vi "Discover Plugins from Loader.vi"(8 "error in (no error)":errorcluster, 10 "Discovery Command":T1, 11 "CIFPluginManager in":refnum<class "CIFPluginManager.lvclass">) -> (0 "error out":errorcluster)   [LabVIEW 2021, in "CIFPluginManager.lvclass"]
uses:
  CIFPluginManager.lvclass
  CIFPluginManager.lvclass/CIFPluginManager.ctl
  CIFCore/Common/Typedef/Version.ctl
  CIFCore/Common/CIFCoreCommon.lvlib
  typedef/Discovered Plugin.ctl
  typedef/Plugin Metadata.ctl
  typedef/Loader Type.ctl
  CIFPluginLoader/gRPC/CIF_Plugin_Loader_Client_Wrapper/CIFPluginLoaderClientWrapper.lvlib
  typedef/Discover Command.ctl
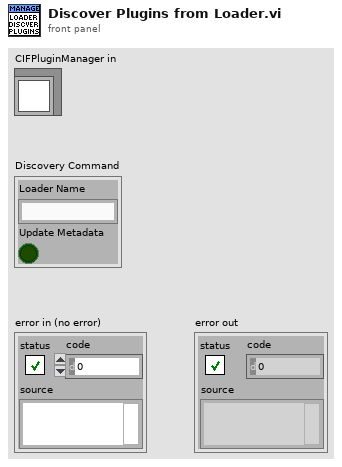
[diagram p1: front panel]
types:
  T1 = typedef "CIFPluginManager.lvclass/Discover Command.ctl" = cluster{"Loader Name":string, "Update Metadata":bool}
  T2 = typedef "CIFPluginManager.lvclass/Loader Map.ctl" = map{string, T3}
  T3 = typedef "CIFPluginManager.lvclass/Loaders.ctl" = cluster{"Loader Type":T4, "grpc_port":i32, "pid":u32, "gRPC ID":T5, "Load Timestamp":i64, "Unloading":bool, "Ready for removal":bool, "Unload Timestamp":i64}
  T4 = typedef "CIFPluginManager.lvclass/Loader Type.ctl" = enum16{"LabVIEW"}
  T5 = typedef "grpc-lvsupport-release.lvlib/grpcId.ctl" = u64
  T6 = typedef "CIFPluginManager.lvclass/Discovered Plugin.ctl" = cluster{"Filename":string, "Plugin Type":string, "Qualified name":string, "Version":T7, "Plugin Metadata":T8, "Loader Type":T4, "File Path":string, "Relative Path":string[]}
  T7 = typedef "CIFCoreCommon.lvlib/Version.ctl" = cluster{"Major":i32, "Minor":i32, "Fix":i32, "Build":i32}
  T8 = typedef "CIFPluginManager.lvclass/Plugin Metadata.ctl" = cluster{"Description":string, "History":string, "Author":string}
  T9 = typedef "CIF_PluginLoader_client.lvlib/cif_pluginloader_DiscoveredPlugin.ctl" = cluster{"file_path":string, "file_name":string, "plugin_type":string, "plugin_version":T10, "plugin_metadata":T11, "relative_path":string[]}
  T10 = typedef "CIF_PluginLoader_client.lvlib/cif_common_Version.ctl" = cluster{"major":u32, "minor":u32, "fix":u32, "build":u32}
  T11 = typedef "CIF_PluginLoader_client.lvlib/cif_manager_PluginMetadata.ctl" = cluster{"description":string, "history":string, "author":string}
  T12 = typedef "CIFPluginManager.lvclass/Discovered Plugin Map.ctl" = map{string, T6[]}
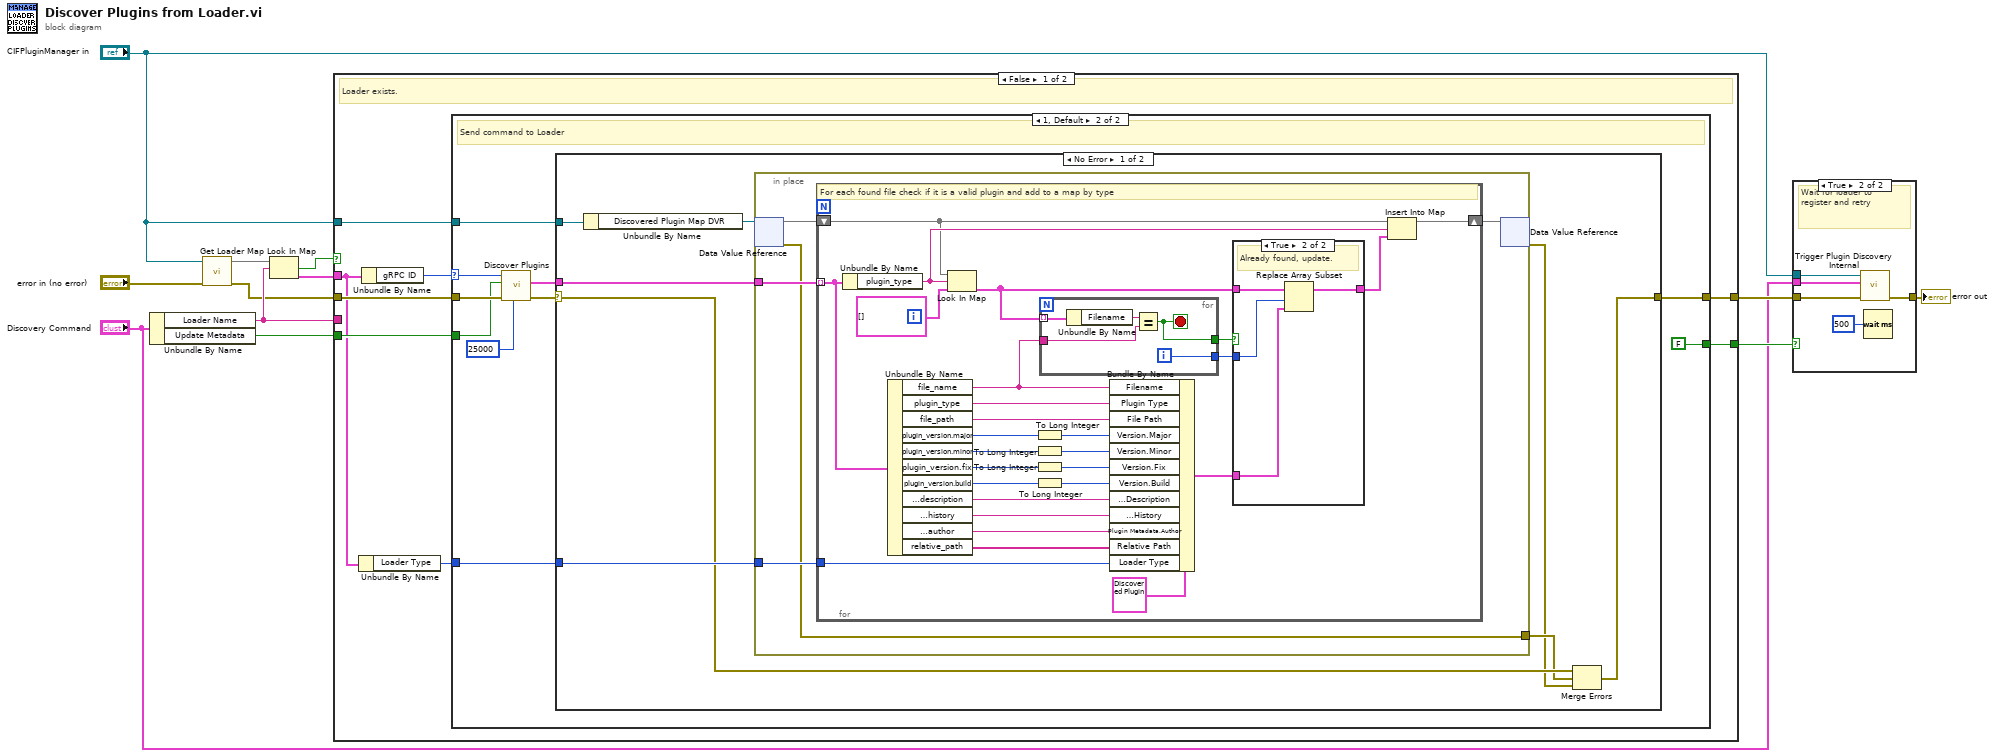
[diagram p0: block diagram]
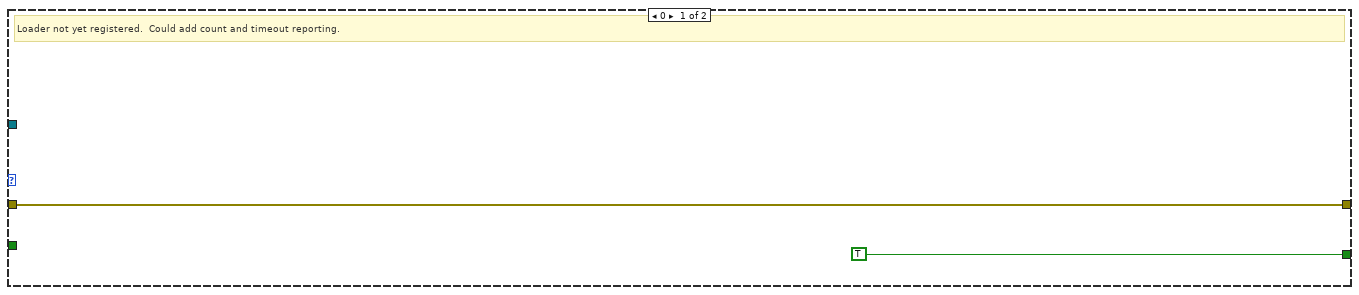
[diagram p3: hidden frame]
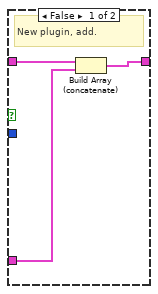
[diagram p4: hidden frame]
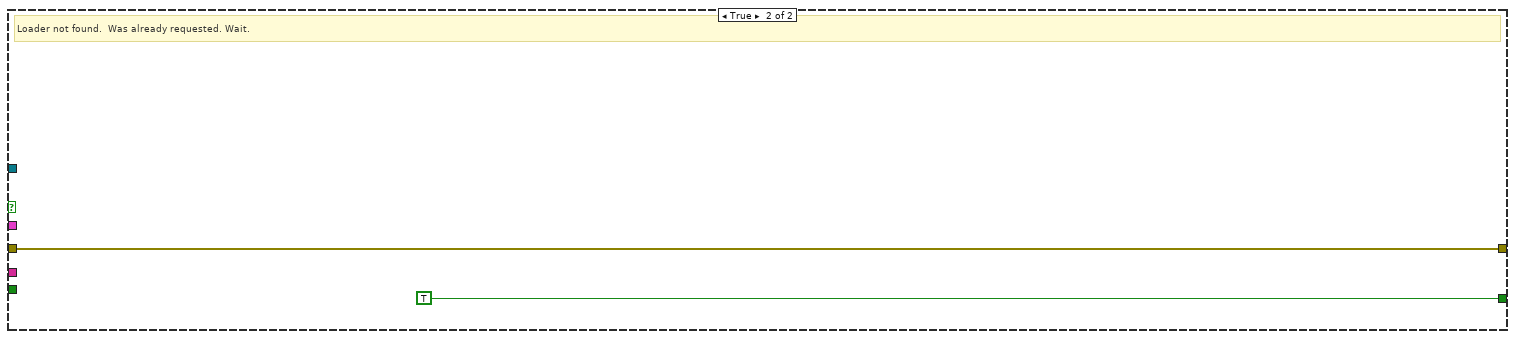
[diagram p6: hidden frame]
diagram:
  n1 = Unbundle By Name("Discovery Command") -> ("Loader Name"=w8:string, "Update Metadata"=w6:bool)
  n2 = call "Get Loader Map.vi"("error in (no error)"="error in (no error)", "CIFPluginManager in"="CIFPluginManager in") -> ("error out"=w3:errorcluster, "Loader Map"=w4:T2)  [unwired: 8 in]
  n3 = Look In Map(map=w4, key=w8) -> (key not found?=w12:bool, value=w10:T3)  [unwired: 1 in]
  n4 = case shown="False" w12 {
    tunnel: "CIFPluginManager in" -> [w16 _]
    tunnel: w3 -> [w17 w86]
    tunnel: [w18 w86] -> w9
    tunnel: w8 -> [_ _]
    tunnel: [w19 TRUE] -> w11
    tunnel: w10 -> [w14 _]
    tunnel: w6 -> [w15 _]
    frame False {
      # "Loader exists."
      n5 = Unbundle By Name(w14) -> ("Loader Type"=w13:T4)
      n6 = Unbundle By Name(w14) -> ("gRPC ID"=w20:T5)
      n7 = case shown="1, Default" w20 {
        selector: w20 -> [_ w32]
        tunnel: [TRUE FALSE] -> w19
        tunnel: [w21 w29] -> w18
        tunnel: w17 -> [w21 w31]
        tunnel: w16 -> [_ w25]
        tunnel: w15 -> [_ w27]
        tunnel: w13 -> [_ w24]
        frame 0 {
          # "Loader not yet registered.  Could add count and timeout reporting."
        }
        frame 1, Default {
          # "Send command to Loader"
          n8 = call "Discover Plugins.vi"("timeout (ms)"=25000, "error in"=w31, "update_metadata"=w27, "gRPC ID in"=w32) -> ("error out"=w28:errorcluster, "discovered_plugins"=w26:T9[])  [unwired: 5 in, 1 out]
          n9 = case shown="No Error" w28 {
            selector: w28 -> [w36 w85]
            tunnel: [w33 w85] -> w29
            tunnel: w26 -> [w39 _]
            tunnel: w25 -> [w40 _]
            tunnel: w24 -> [w38 _]
            frame No Error {
              n10 = Unbundle By Name(w40) -> ("Discovered Plugin Map DVR"=w37:refnum<data-value>)
              n11 = in-place {
                in-place-border: w39 -> [w45]
                in-place-border: w38 -> [w44]
                in-place-border: [w41] -> w35
                n12 = in-place-dvr #1(w37) -> (w43:T12, w41:errorcluster)
                n13 = for {
                  tunnel: w45 -> [w62] mode=indexing
                  shift-right: [w65] -> w42
                  shift-left: w43 -> [w66]
                  tunnel: w44 -> [w47]
                  # "For each found file check if it is a valid plugin and add to a map by type"
                  n14 = Unbundle By Name(w62) -> ("plugin_type"=w67:string)
                  n15 = Unbundle By Name(w62) -> ("file_name"=w61:string, "plugin_type"=w60:string, "file_path"=w59:string, "plugin_version.major"=w48:u32, "plugin_version.minor"=w49:u32, "plugin_version.fix"=w58:u32, "plugin_version.build"=w57:u32, "plugin_metadata.description"=w52:string, "plugin_metadata.history"=w51:string, "plugin_metadata.author"=w50:string, "relative_path"=w46:string[])
                  n16 = Look In Map(map=w66, key=w67, default value=T6[] [] ("value")) -> (value=w70:T6[])  [unwired: 1 out]
                  n17 = To Long Integer(number=w48) -> (32bit integer=w56:i32)
                  n18 = To Long Integer(number=w49) -> (32bit integer=w55:i32)
                  n19 = To Long Integer(number=w58) -> (32bit integer=w54:i32)
                  n20 = To Long Integer(number=w57) -> (32bit integer=w53:i32)
                  n21 = for {
                    tunnel: w61 -> [w83]
                    tunnel: w70 -> [w80] mode=indexing
                    tunnel: [w82] -> w71
                    tunnel: [w81] -> w69
                    i -> [w81]
                    stop <- w82 stop-if-true
                    n22 = Unbundle By Name(w80) -> ("Filename"=w84:string)
                    n23 = Equal?(x=w84, y=w83) -> (x = y?=w82:bool)
                  }
                  n24 = Bundle By Name(cluster=T6 {"Filename"="", "Plugin Type"="", "Qualified name"="", "Version"={"Major"=0, "Minor"=0, "Fix"=0, "Build"=0}, "Plugin Metadata"={"Description"="", "History"="", "Author"=""}, "Loader Type"=enum."LabVIEW", "File Path"="", "Relative Path"=[]} ("Discovered Plugin"), "Filename"=w61, "Plugin Type"=w60, "File Path"=w59, "Version.Major"=w56, "Version.Minor"=w55, "Version.Fix"=w54, "Version.Build"=w53, "Plugin Metadata.Description"=w52, "Plugin Metadata.History"=w51, "Plugin Metadata.Author"=w50, "Relative Path"=w46, "Loader Type"=w47) -> (w64:T6)
                  n25 = case shown="True" w71 {
                    tunnel: w64 -> [w74 w79]
                    tunnel: w70 -> [w75 w78]
                    tunnel: [w73 w76] -> w68
                    tunnel: w69 -> [_ w77]
                    frame False {
                      # "New plugin, add."
                      n26 = Build Array (concatenate)(w75, w74) -> (w73:T6[])
                    }
                    frame True {
                      # "Already found, update."
                      n27 = Replace Array Subset(array=w78, new element=w79, index=w77) -> (w76:T6[])
                    }
                  }
                  n28 = Insert Into Map(map in=w66, key=w67, value=w68) -> (map out=w65:T12)  [unwired: 2 out]
                }
                n29 = in-place-dvr #1(w42) -> (w34:errorcluster)  [unwired: 1 out]
              }
              n30 = Merge Errors(w36, w35, w34) -> (w33:errorcluster)
            }
            frame Error {
            }
          }
        }
      }
    }
    frame True {
      # "Loader not found.  Was already requested. Wait."
    }
  }
  n31 = case shown="True" w11 {
    tunnel: w9 -> [w88 w90]
    tunnel: "CIFPluginManager in" -> [_ w92]
    tunnel: "Discovery Command" -> [_ w91]
    tunnel: [w88 w89] -> w2
    frame False {
    }
    frame True {
      # "Wait for loader to register and retry"
      n32 = call "Trigger Plugin Discovery Internal.vi"("error in (no error)"=w90, "Trigger Discovery"=w91, "CIFPluginManager in"=w92) -> ("error out"=w89:errorcluster)  [unwired: 8 in]
      n33 = Wait (ms)(milliseconds to wait=u32 500) -> ()  [unwired: 1 out]
    }
  }
  "error out" <- w2
